vi "Main - Separate File and Output sessions - UEIDAQ Only.vi"() -> ()   [LabVIEW 2012]
uses:
  ChannelStateControl.ctl
  <vilib>/UeiDaq/UeiDaqCreateDOSession.vi
  <vilib>/UeiDaq/UeiDaqConfigureTimingForSimpleIO.vi
  <vilib>/UeiDaq/UeiDaqWriteDigitalDataUInt16.vi
  <vilib>/UeiDaq/UeiDaqWriteOneDigitalScanUInt16.vi
  <resource>/objmgr/UeiDaq.rc
panel:
  out "Timing Changed?":bool
  in  "#DIO Ports (Adjustable)":u32
  out "Initial States":u16[](array[numeric])
  in  "DIO Groups":T1[](array[typedef])=[{"Channel 1"=0, "Enable"=TRUE, "Main Switch"=0, "Channel 2"=0, "Channel 9"=0, "Channel 10"=0, "Channel 11"=0, "Channel 3"=0, "Channel 4"=0, "Channel 12"=0, "Channel 5"=0, "Channel 13"=0, "Channel 6"=0, "Channel 14"=0, "Channel 7"=0, "Channel 15"=0, "Channel 8"=0, "Channel 16"=0}, {"Channel 1"=0, "Enable"=TRUE, "Main Switch"=0, "Channel 2"=0, "Channel 9"=0, "Channel 10"=0, "Channel 11"=0, "Channel 3"=0, "Channel 4"=0, "Channel 12"=0, "Channel 5"=0, "Channel 13"=0, "Channel 6"=0, "Channel 14"=0, "Channel 7"=0, "Channel 15"=0, "Channel 8"=0, "Channel 16"=0}, {"Channel 1"=0, "Enable"=TRUE, "Main Switch"=0, "Channel 2"=0, "Channel 9"=0, "Channel 10"=0, "Channel 11"=0, "Channel 3"=0, "Channel 4"=0, "Channel 12"=0, "Channel 5"=0, "Channel 13"=0, "Channel 6"=0, "Channel 14"=0, "Channel 7"=0, "Channel 15"=0, "Channel 8"=0, "Channel 16"=0}, {"Channel 1"=0, "Enable"=TRUE, "Main Switch"=0, "Channel 2"=0, "Channel 9"=0, "Channel 10"=0, "Channel 11"=0, "Channel 3"=0, "Channel 4"=0, "Channel 12"=0, "Channel 5"=0, "Channel 13"=0, "Channel 6"=0, "Channel 14"=0, "Channel 7"=0, "Channel 15"=0, "Channel 8"=0, "Channel 16"=0}, {"Channel 1"=0, "Enable"=TRUE, "Main Switch"=0, "Channel 2"=0, "Channel 9"=0, "Channel 10"=0, "Channel 11"=0, "Channel 3"=0, "Channel 4"=0, "Channel 12"=0, "Channel 5"=0, "Channel 13"=0, "Channel 6"=0, "Channel 14"=0, "Channel 7"=0, "Channel 15"=0, "Channel 8"=0, "Channel 16"=0}, {"Channel 1"=0, "Enable"=TRUE, "Main Switch"=0, "Channel 2"=0, "Channel 9"=0, "Channel 10"=0, "Channel 11"=0, "Channel 3"=0, "Channel 4"=0, "Channel 12"=0, "Channel 5"=0, "Channel 13"=0, "Channel 6"=0, "Channel 14"=0, "Channel 7"=0, "Channel 15"=0, "Channel 8"=0, "Channel 16"=0}]
  out "Quantum Composer Command":string[](array[string])
  out "Main Loop Stopped?":bool
  out "Status Indicator":bool[][](array[boolean])
  out "Total Step":u64
  out "Original Timing Signal":i16[][](array[numeric]) format="%b"
  out "Running":bool
  in  "DIO Port":string="pwrdaq://Dev0/Do0:2"
  in  "stop":bool
  out "Loop Count":i32
  in  "Loop":bool
  out "Parsed File Location":path
  in  "All Low":bool
  in  "Run":bool
  in  "Timing Array (Adjustable)":i32[](array[numeric])=[0, 0, 0, 0, 0, 0, 0, 0, 0, 0, 0, 0, 0, 0, 0, 0, 0, 0, 0, 0] caption="Timing Array (Time Duration for each signal)"
  in  "Modified Timing Signal":i16[][](array[numeric])=[[0, 0, 0, 0, 0, 0, 0, 0, 0, 0, 0, 0, 0, 0, 0, 0, 0, 0, 0, 0]] caption="Modified Timing Signal (after adjustment from I/O channel panel)" format="%b"
  in  "Compile and Load":bool
  out "Channel Names":string[](array[string])
  out "Channel Number":u16=48
  in  "Timing File":path
  in  "Perl Parser":path=path "C:/Labview/Parser File/parse-timing.pl"
  # "(Use Do0:5 for DIO0-DIO5, 6ch,  Do0;5 for DIO0 and DIO5, 2ch)"
  # "Control Panel"
  # "(pwrdaq://Dev0 for real I/O; simu://Dev2 for simulated DAQ card)"
  # "1"
  # "2"
  # "3"
  # "4"
  # "5"
  # "6"
  # "7"
  # "8"
  # "9"
  # "10"
  # "11"
  # "12"
  # "13"
  # "14"
  # "15"
  # "16"
  # "Group1"
  # "Group2"
  # "Group3"
  # "Group4"
  # "Group5"
  # "Group6"
  # "(Currently, When \"STOP Loop\" is pressed, the status remain in the final state, when ER stop is pressed, all channels will be set as \"low\")"
  # "Status Panel"
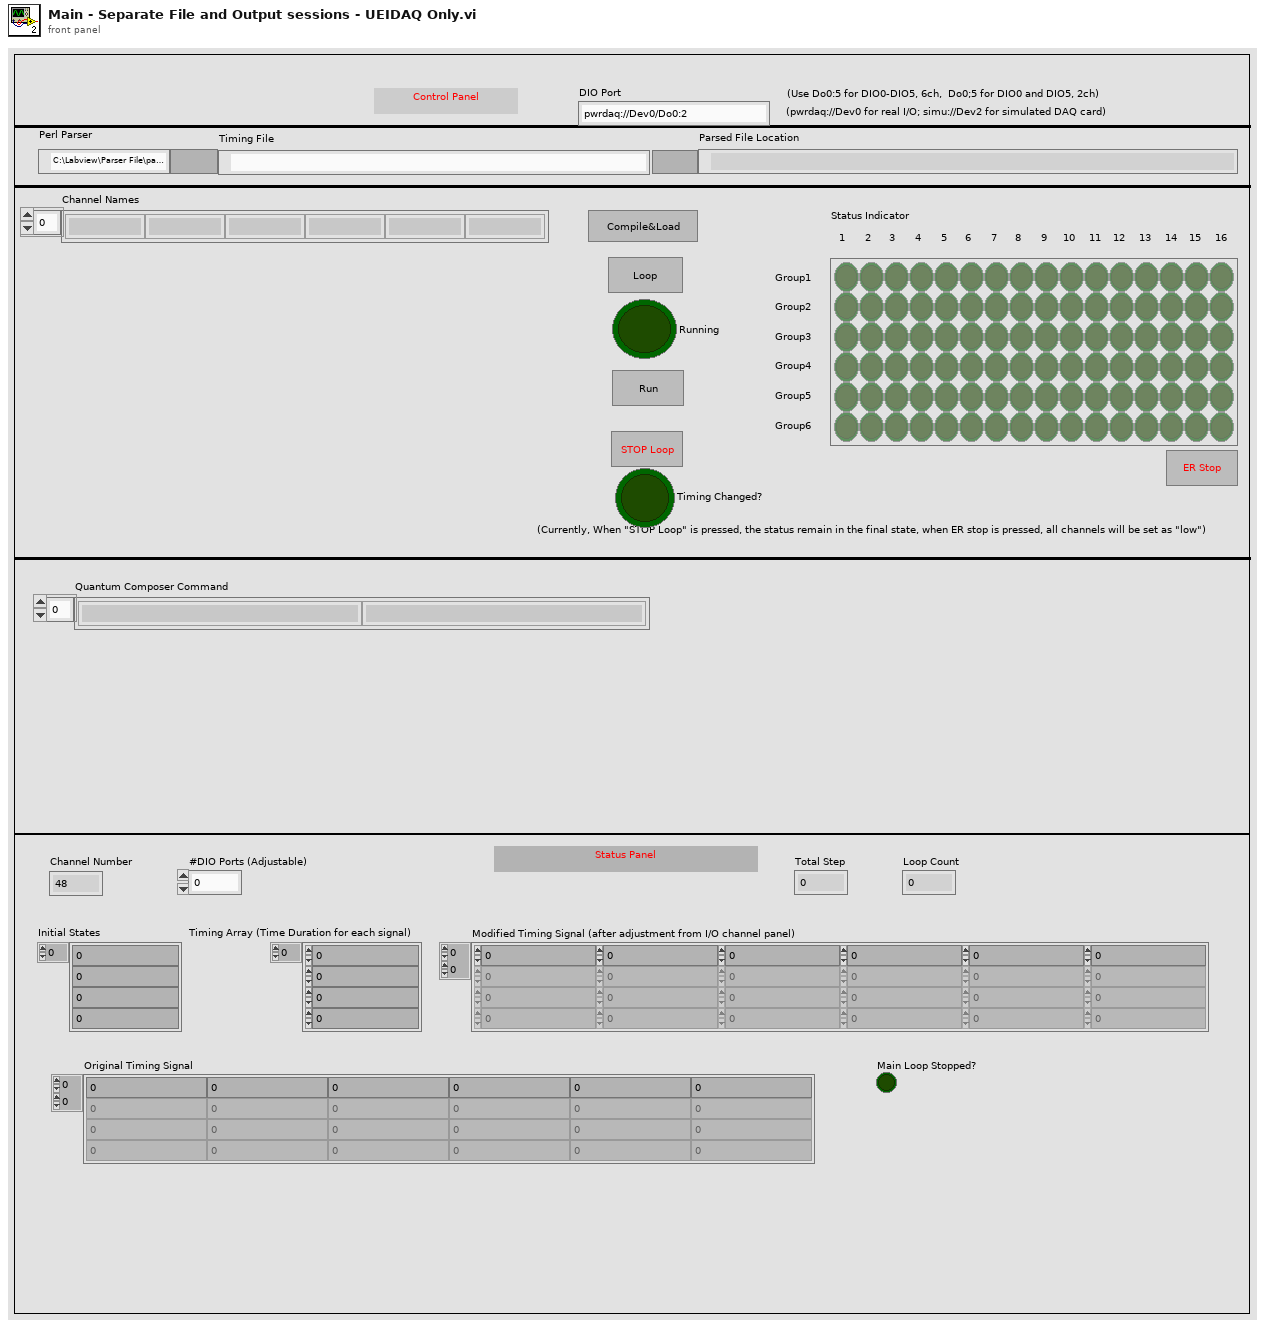
[diagram p1: front panel]
types:
  T1 = typedef "ChannelStateControl.ctl" = cluster{"Channel 1":u8, "Enable":bool, "Main Switch":u8, "Channel 2":u8, "Channel 9":u8, "Channel 10":u8, "Channel 11":u8, "Channel 3":u8, "Channel 4":u8, "Channel 12":u8, "Channel 5":u8, "Channel 13":u8, "Channel 6":u8, "Channel 14":u8, "Channel 7":u8, "Channel 15":u8, "Channel 8":u8, "Channel 16":u8}
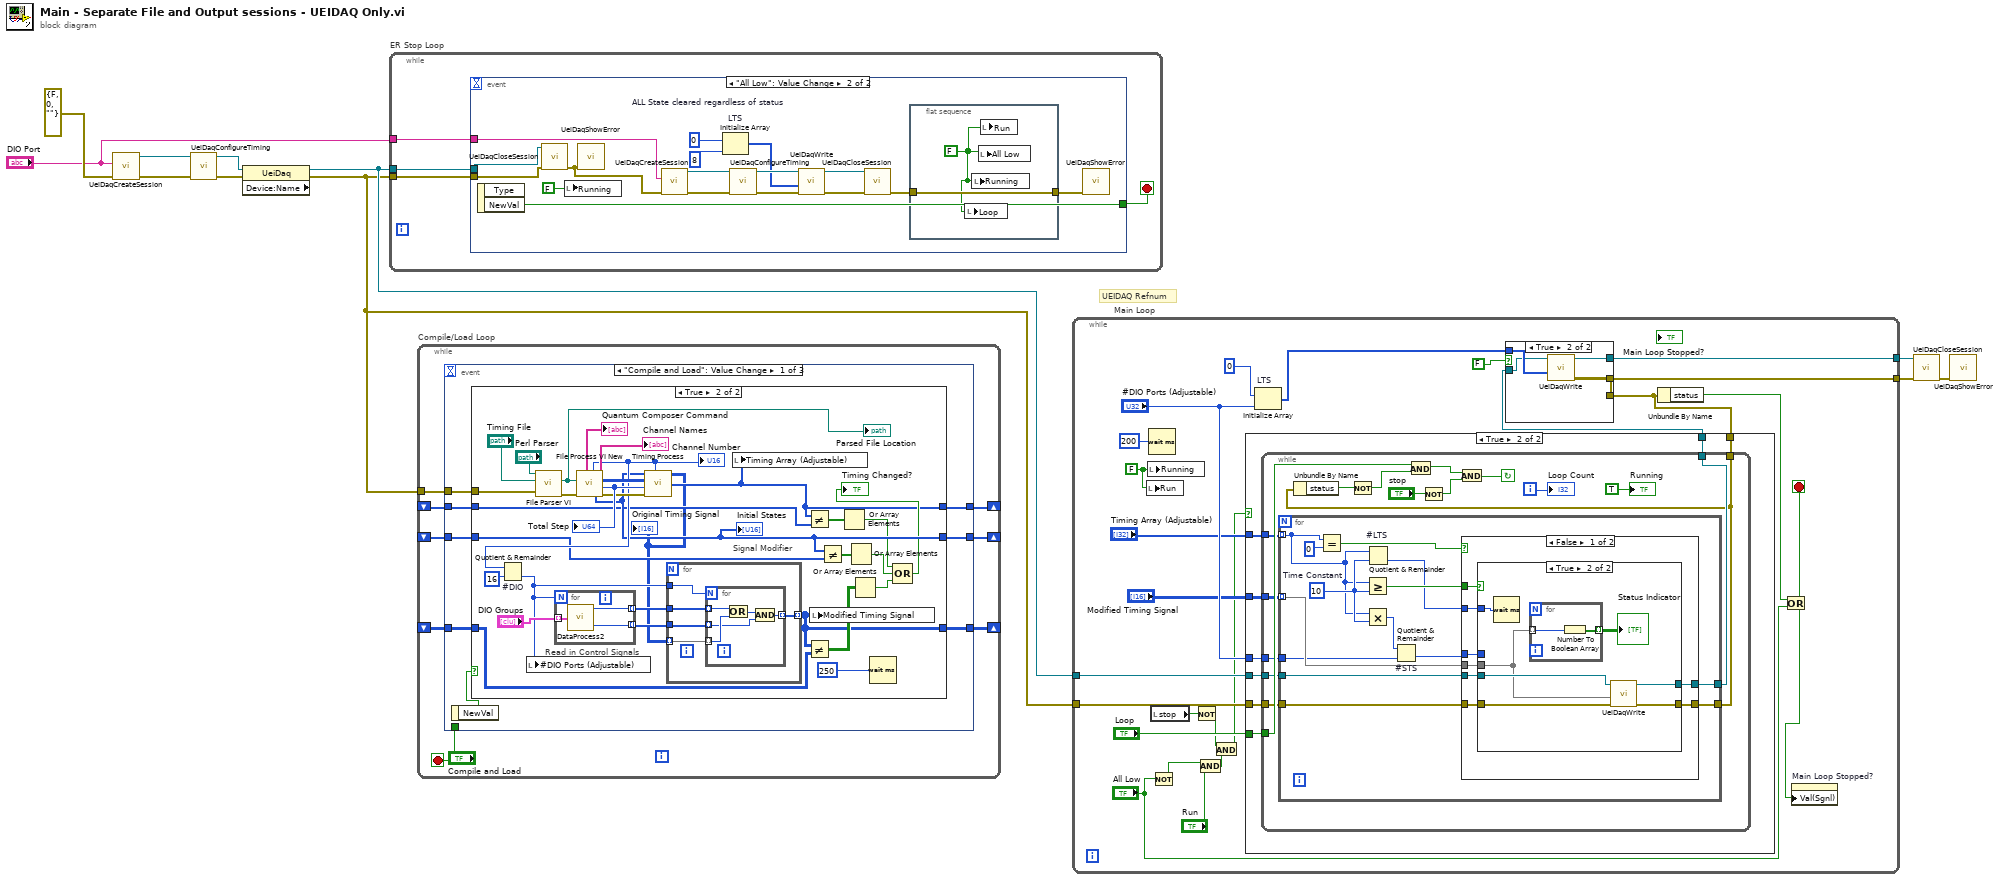
[diagram p0: block diagram]
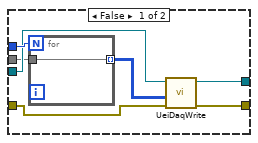
[diagram p4: hidden frame]
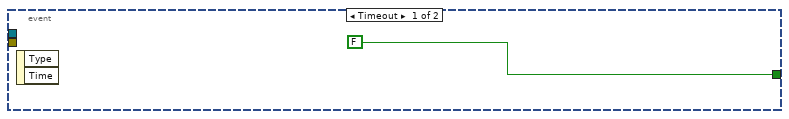
[diagram p6: hidden frame]
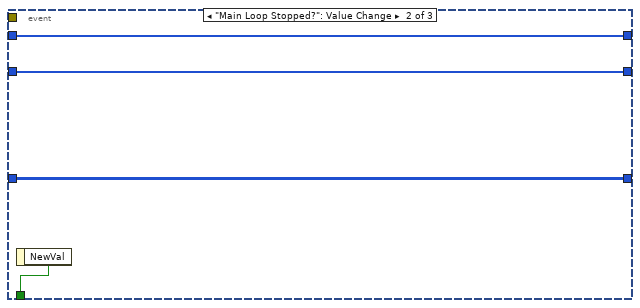
[diagram p8: hidden frame]
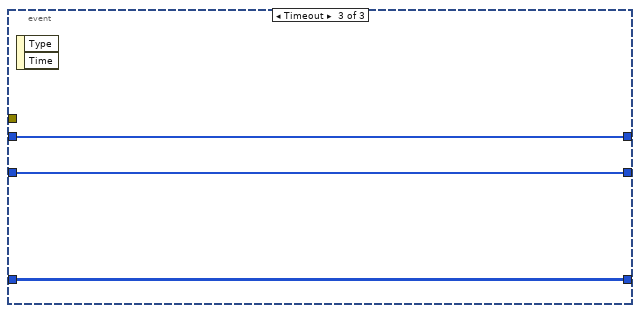
[diagram p9: hidden frame]
diagram:
  # "UEIDAQ Refnum"
  n1 = call-poly <vilib>:"UeiDaqCreateSession.vi"("error in (no error)"=errorcluster {"status"=FALSE, "code"=0, "source"=""} ("error constant"), "Resource"="DIO Port") -> ("error out"=w10:errorcluster, "UeiDaq Refnum Out"=w11:refnum<k20>)  [unwired: 8 in]
  n2 = call-poly <vilib>:"UeiDaqConfigureTiming.vi"("error in (no error)"=w10, "UeiDaq Refnum In"=w11) -> ("error out"=w8:errorcluster, "UeiDaq Refnum Out"=w9:refnum<k20>)  [unwired: 8 in]
  n3 = property class="UeiDaq" props=["Device:Name"](reference=w9, error in=w8) -> (reference out=w4:refnum<k20>, error out=w3:errorcluster)  [unwired: 1 out]
  n4 = while "ER Stop Loop" {
    tunnel: w3 -> [w14]
    tunnel: w4 -> [w13]
    tunnel: "DIO Port" -> [w12]
    stop <- w15 stop-if-true
    n5 = event shown="[1] \"All Low\": Value Change" {
      selector: _ -> [_ _]
      dyn-events: _ -> [_ _]
      timeout: _ -> [_ _]
      tunnel: [FALSE w33] -> w15
      tunnel: w14 -> [_ w31]
      tunnel: w13 -> [_ w32]
      tunnel: w12 -> [_ w17]
      event Timeout {
        n6 = event-data() -> ()  [unwired: 1 in, 2 out]
      }
      event "All Low": Value Change {
        w22 = 8  # ALL State cleared regardless of status
        n7 = event-data() -> ("NewVal"=w33:bool)  [unwired: 1 in, 1 out]
        n8 = call <vilib>:"UeiDaqCloseSession.vi"("error in (no error)"=w31, "UeiDaq Refnum In"=w32) -> ("error out"=w18:errorcluster)  [unwired: 8 in, 1 out]
        n9 = local write "Running"(FALSE) -> ()
        n10 = call <vilib>:"UeiDaqShowError.vi"("error in (no error)"=w18) -> ()  [unwired: 10 in, 1 out]
        n11 = call-poly <vilib>:"UeiDaqCreateSession.vi"("error in (no error)"=w18, "Resource"=w17) -> ("error out"=w25:errorcluster, "UeiDaq Refnum Out"=w24:refnum<k20>)  [unwired: 8 in]
        n12 = Initialize Array "LTS"(i16 0, w22) -> (w23:i16[])
        n13 = call-poly <vilib>:"UeiDaqConfigureTiming.vi"("error in (no error)"=w25, "UeiDaq Refnum In"=w24) -> ("error out"=w27:errorcluster, "UeiDaq Refnum Out"=w26:refnum<k20>)  [unwired: 8 in]
        n14 = call-poly <vilib>:"UeiDaqWrite.vi"("error in (no error)"=w27, "Digital Data"=w23, "UeiDaq Refnum In"=w26) -> ("error out"=w20:errorcluster, "UeiDaq Refnum Out"=w19:refnum<k20>)  [unwired: 7 in]
        n15 = call <vilib>:"UeiDaqCloseSession.vi"("error in (no error)"=w20, "UeiDaq Refnum In"=w19) -> ("error out"=w29:errorcluster)  [unwired: 8 in, 1 out]
        n16 = flat-sequence {
          tunnel: [w35] -> w28
          tunnel: w29 -> [w35]
          frame #0 {
            w34 = FALSE
            n17 = local write "Loop"(w34) -> ()
            n18 = local write "Running"(w34) -> ()
            n19 = local write "All Low"(w34) -> ()
            n20 = local write "Run"(w34) -> ()
          }
        }
        n21 = call <vilib>:"UeiDaqShowError.vi"("error in (no error)"=w28) -> ()  [unwired: 10 in, 1 out]
      }
    }
  }
  n22 = while "Compile/Load Loop" {
    tunnel: w3 -> [w43]
    shift-right: [w41] -> _
    shift-left: _ -> [w38]
    shift-right: [w40] -> _
    shift-left: _ -> [w36]
    shift-right: [w39] -> _
    shift-left: _ -> [w37]
    stop <- w42 stop-if-true
    n23 = event shown="[0] \"Compile and Load\": Value Change" {
      selector: _ -> [_ _ _]
      dyn-events: _ -> [_ _ _]
      timeout: _ -> [_ _ _]
      tunnel: w43 -> [w51 _ _]
      tunnel: [_ w102 _] -> w42
      tunnel: [w49 w101 w105] -> w41
      tunnel: [w48 w99 w103] -> w40
      tunnel: [w47 w100 w104] -> w39
      tunnel: w38 -> [w46 w101 w105]
      tunnel: w37 -> [w45 w100 w104]
      tunnel: w36 -> [w44 w99 w103]
      event "Compile and Load": Value Change {
        n24 = event-data() -> ("NewVal"=w50:bool)  [unwired: 1 in]
        n25 = case shown="True" w50 {
          tunnel: w51 -> [_ w74]
          tunnel: [w54 w57] -> w49
          tunnel: [w52 w64] -> w48
          tunnel: [w53 w67] -> w47
          tunnel: w46 -> [w54 w56]
          tunnel: w45 -> [w53 w66]
          tunnel: w44 -> [w52 w63]
          frame False {
          }
          frame True {
            n26 = call "File Parser VI.vi"("error in (no error)"=w74, "Original Timing File Path"="Timing File", "Perl Parser Path"="Perl Parser") -> ("error out"=w83:errorcluster, "Parsed File Path"=w81:path)  [unwired: 7 in]
            "Parsed File Location" <- w81
            n27 = call "File Process VI New.vi"("error in (no error)"=w83, "Parsed File Path"=w81) -> ("Error Out"=w73:errorcluster, "Total Step"=w79:u64, "Switching Times"=w80:u32[][], "Channel Names"=→"Channel Names":string[], "Initial States"=w67:u16[], "Channel Number"=w71:u16, "GPIB Output"=→"Quantum Composer Command":string[])  [unwired: 3 in]
            "Channel Number" <- w71
            "Total Step" <- w79
            "Initial States" <- w67
            n28 = Quotient & Remainder "#DIO"(x=w71, y=u16 16) -> (floor(x/y)=w58:u16)  [unwired: 1 out]
            n29 = local write "#DIO Ports (Adjustable)"(w58) -> ()
            n30 = for "Read in Control Signals" {
              N: w58 -> [_]
              tunnel: "DIO Groups" -> [w88] mode=indexing
              tunnel: [w87] -> w77 mode=indexing
              tunnel: [w86] -> w76 mode=indexing
              n31 = call "DataProcess2.vi"("DIO Group 1"=w88) -> ("High"=w87:u16, "Low"=w86:u16)
            }
            n32 = call "Timing Process.vi"("Initial States"=w67, "Switching Times"=w80, "Total Steps"=w79, "error in (no error)"=w73, "Channel"=w71) -> ("Output Signal Array"=w55:i16[][], "Output Time Array"=w57:i32[])  [unwired: 1 out]
            "Original Timing Signal" <- w55
            n33 = for "Signal Modifier" {
              tunnel: w55 -> [w93] mode=indexing
              tunnel: [w92] -> w64 mode=indexing
              tunnel: w77 -> [w91]
              tunnel: w76 -> [w90]
              tunnel: w58 -> [w89]
              n34 = for {
                N: w89 -> [_]
                tunnel: w93 -> [w98] mode=indexing
                tunnel: [w96] -> w92 mode=indexing
                tunnel: w91 -> [w95] mode=indexing
                tunnel: w90 -> [w94] mode=indexing
                n35 = Or(x=w95, y=w98) -> (x .or. y?=w97:u16)
                n36 = And(x=w97, y=w94) -> (x .and. y?=w96:u16)
              }
            }
            n37 = local write "Timing Array (Adjustable)"(w57) -> ()
            n38 = Not Equal?(x=w57, y=w56) -> (x != y?=w69:bool[])
            n39 = Not Equal?(x=w64, y=w63) -> (x != y?=w65:bool[][])
            n40 = local write "Modified Timing Signal"(w64) -> ()
            n41 = Not Equal?(x=w67, y=w66) -> (x != y?=w68:bool[])
            n42 = Or Array Elements(Boolean array=w69) -> (logical OR=w62:bool)
            n43 = Or Array Elements(Boolean array=w68) -> (logical OR=w61:bool)
            n44 = Or Array Elements(Boolean array=w65) -> (logical OR=w60:bool)
            n45 = Wait (ms)(milliseconds to wait=250) -> ()  [unwired: 1 out]
            n46 = Compound Arithmetic op=OR(w62, w61, w60) -> (→"Timing Changed?":bool)
          }
        }
      }
      event "Main Loop Stopped?": Value Change {
        n47 = event-data() -> ("NewVal"=w102:bool)  [unwired: 1 in]
      }
      event Timeout {
        n48 = event-data() -> ()  [unwired: 1 in, 2 out]
      }
    }
  }
  n49 = while "Main Loop" {
    tunnel: w4 -> [w119]
    tunnel: w3 -> [w117]
    tunnel: [w115] -> w2
    tunnel: [w114] -> w1
    stop <- w118 stop-if-true
    w121 = FALSE
    n50 = local write "Run"(w121) -> ()
    n51 = local write "Running"(w121) -> ()
    n52 = Wait (ms)(milliseconds to wait=200) -> ()  [unwired: 1 out]
    n53 = local read "stop"() -> (w109:bool)
    n54 = Not(x="All Low") -> (.not. x?=w129:bool)
    n55 = Not(x=w109) -> (.not. x?=w108:bool)
    n56 = And(x=w129, y="Run") -> (x .and. y?=w111:bool)
    n57 = And(x=w108, y=w111) -> (x .and. y?=w110:bool)
    n58 = case shown="True" w110 {
      tunnel: "Loop" -> [_ w146]
      tunnel: [w137 w145] -> w127
      tunnel: [w138 w144] -> w126
      tunnel: w119 -> [w138 w143]
      tunnel: w117 -> [w137 w142]
      tunnel: "Timing Array (Adjustable)" -> [_ w141]
      tunnel: "Modified Timing Signal" -> [_ w140]
      tunnel: "#DIO Ports (Adjustable)" -> [_ w139]
      frame False {
      }
      frame True {
        n59 = while {
          tunnel: w146 -> [w155]
          tunnel: [w156] -> w145
          tunnel: [w162] -> w144
          tunnel: w143 -> [w151]
          tunnel: w142 -> [w150]
          tunnel: w141 -> [w149]
          tunnel: w140 -> [w148]
          tunnel: w139 -> [w147]
          i -> [w161]
          stop <- w159 continue-if-true
          n60 = for {
            tunnel: [w175] -> w156
            tunnel: [w173] -> w162
            tunnel: w151 -> [w167]
            tunnel: w150 -> [w166]
            tunnel: w149 -> [w163] mode=indexing
            tunnel: w148 -> [w165] mode=indexing
            tunnel: w147 -> [w164]
            w168 = 10  # Time Constant
            n61 = Equal?(x=w163, y=0) -> (x = y?=w171:bool)
            n62 = Greater Or Equal?(x=w163, y=w168) -> (x >= y?=w176:bool)
            n63 = Multiply(x=w163, y=w168) -> (x*y=w170:i32)
            n64 = Quotient & Remainder "#LTS"(x=w163, y=w168) -> (floor(x/y)=w174:i32)  [unwired: 1 out]
            n65 = Quotient & Remainder "#STS"(x=w170, y=w164) -> (floor(x/y)=w169:u32)  [unwired: 1 out]
            n66 = case shown="False" w171 {
              tunnel: w176 -> [w184 _]
              tunnel: [w183 w202] -> w175
              tunnel: w174 -> [w182 _]
              tunnel: [w181 w203] -> w173
              tunnel: w169 -> [w180 _]
              tunnel: w167 -> [w179 w203]
              tunnel: w166 -> [w178 w202]
              tunnel: w165 -> [w177 _]
              frame False {
                n67 = case shown="True" w184 {
                  tunnel: [w191 w199] -> w183
                  tunnel: w182 -> [_ w198]
                  tunnel: [w190 w197] -> w181
                  tunnel: w180 -> [w189 _]
                  tunnel: w179 -> [w188 w195]
                  tunnel: w178 -> [w187 w194]
                  tunnel: w177 -> [w185 w193]
                  frame False {
                    n68 = for {
                      N: w189 -> [_]
                      tunnel: [w192] -> w186 mode=indexing
                      tunnel: w185 -> [w192]
                    }
                    n69 = call-poly <vilib>:"UeiDaqWrite.vi"("error in (no error)"=w187, "Digital Data"=w186, "UeiDaq Refnum In"=w188) -> ("error out"=w191:errorcluster, "UeiDaq Refnum Out"=w190:refnum<k20>)  [unwired: 7 in]
                  }
                  frame True {
                    n70 = Wait (ms)(milliseconds to wait=w198) -> ()  [unwired: 1 out]
                    n71 = for {
                      tunnel: [w201] -> w196 mode=indexing
                      tunnel: w193 -> [w200] mode=indexing
                      n72 = Number To Boolean Array(number=w200) -> (Boolean array=w201:bool[])
                    }
                    "Status Indicator" <- w196
                    n73 = call-poly <vilib>:"UeiDaqWrite.vi"("error in (no error)"=w194, "Digital Data"=w193, "UeiDaq Refnum In"=w195) -> ("error out"=w199:errorcluster, "UeiDaq Refnum Out"=w197:refnum<k20>)  [unwired: 7 in]
                  }
                }
              }
              frame True {
              }
            }
          }
          n74 = Unbundle By Name(w156) -> ("status"=w157:bool)
          n75 = Not(x=w157) -> (.not. x?=w154:bool)
          n76 = And(x=w155, y=w154) -> (x .and. y?=w153:bool)
          n77 = Not(x="stop") -> (.not. x?=w152:bool)
          n78 = And(x=w153, y=w152) -> (x .and. y?=w159:bool)
          "Loop Count" <- w161
          "Running" <- TRUE
        }
      }
    }
    n79 = Initialize Array "LTS"(i16 0, "#DIO Ports (Adjustable)") -> (w125:i16[])
    n80 = case shown="True" FALSE {
      tunnel: w125 -> [_ w136]
      tunnel: w126 -> [w131 w135]
      tunnel: [w131 w134] -> w115
      tunnel: w127 -> [w130 w133]
      tunnel: [w130 w132] -> w114
      frame False {
      }
      frame True {
        n81 = call-poly <vilib>:"UeiDaqWrite.vi"("error in (no error)"=w133, "Digital Data"=w136, "UeiDaq Refnum In"=w135) -> ("error out"=w132:errorcluster, "UeiDaq Refnum Out"=w134:refnum<k20>)  [unwired: 7 in]
      }
    }
    n82 = Unbundle By Name(w127) -> ("status"=w123:bool)
    n83 = Or(x=w123, y="All Low") -> (x .or. y?=w118:bool)
    n84 = property on="Main Loop Stopped?" class="Bool (strict)"("Val(Sgnl)"=w118) -> ()  [unwired: 2 in, 2 out]
  }
  n85 = call <vilib>:"UeiDaqCloseSession.vi"("error in (no error)"=w1, "UeiDaq Refnum In"=w2) -> ("error out"=w6:errorcluster)  [unwired: 8 in, 1 out]
  n86 = call <vilib>:"UeiDaqShowError.vi"("error in (no error)"=w6) -> ()  [unwired: 10 in, 1 out]
